vi "tsdiag_clear_diagnostic_information.vi"(7 "DTC descriptor":T1={"DTC Byte Length"=3, "Status Byte Length"=1, "Add Data Byte Length"=0, "Byte Order"=enum."Motorola"}, 8 "error in (no error)":errorcluster, 9 "group of DTC":u32=16777215 format="%.0x", 10 "ADiagModuleIndex":i32, 11 "path":path) -> (0 "error out":errorcluster, 1 "success?":bool, 2 "Return Type":i32, 3 "path out":path)   [LabVIEW 2014]
doc: "14服务，清除诊断信息。"
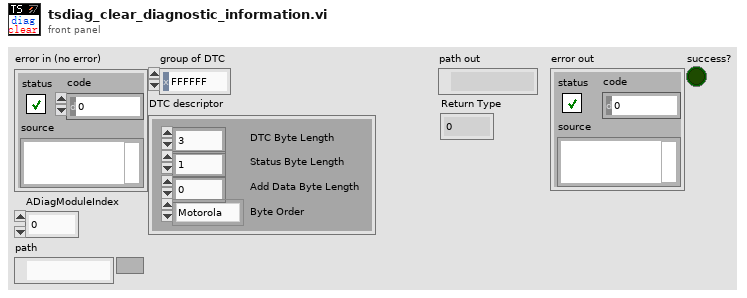
[diagram p1: front panel]
types:
  T1 = cluster{"DTC Byte Length":i32, "Status Byte Length":i32, "Add Data Byte Length":i32, "Byte Order":enum16{"Motorola", "Intel"}}
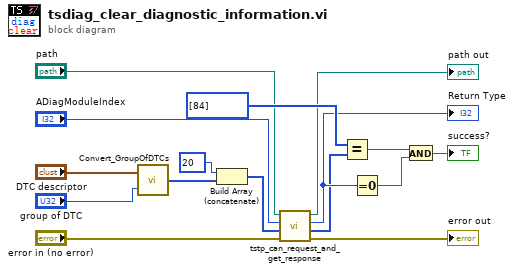
[diagram p0: block diagram]
diagram:
  n1 = call "Convert_GroupOfDTCs.vi"("group of DTC"="group of DTC", "DTC descriptor"="DTC descriptor") -> ("data out"=w10:u8[])
  n2 = Build Array (concatenate)(u8 20 ("element"), w10) -> (w6:u8[])
  n3 = call "tstp_can_request_and_get_response.vi"("错误输入（无错误）"="error in (no error)", "AReqDataArray"=w6, "ADiagModuleIndex"="ADiagModuleIndex", "path"="path") -> ("错误输出"=→"error out":errorcluster, "Diagnostic response"=w1:u8[], "Return Type"=w3:i32, "path out"=→"path out":path)  [unwired: 4 in]
  "Return Type" <- w3
  n4 = Equal?(x=u8[] [84], y=w1) -> (x = y?=w15:bool)
  n5 = Equal To 0?(x=w3) -> (x = 0?=w2:bool)
  n6 = And(x=w15, y=w2) -> (x .and. y?=→"success?":bool)
